vi "MBUS_U8toU16.vi"(11 "inputData":u8[](array[numeric])) -> (2 "ModbusExceptionCode":u8, 3 "outputData":u16[](array[numeric]))   [LabVIEW 2012, in "MBUS_Modbus.lvlib"]
uses:
  MBUS_Modbus.lvlib
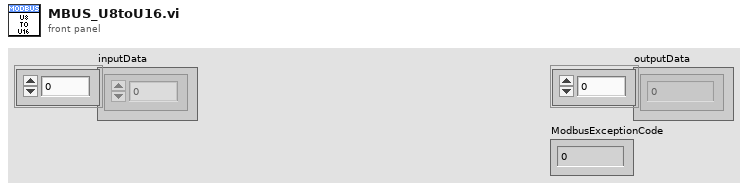
[diagram p1: front panel]
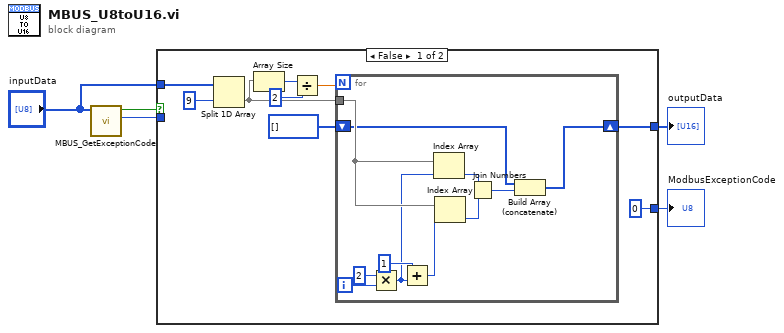
[diagram p0: block diagram]
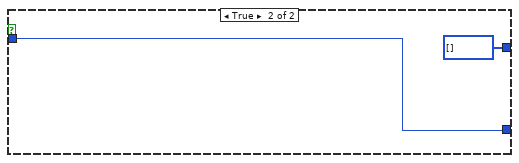
[diagram p2: hidden frame]
diagram:
  n1 = call "MBUS_GetExceptionCode.vi"("inputData"="inputData") -> ("ModbusExceptionCode"=w4:u8, "ModbusException"=w5:bool)  [unwired: 9 in]
  n2 = case shown="False" w5 {
    tunnel: w4 -> [_ w26]
    tunnel: "inputData" -> [w14 _]
    tunnel: [w11 u16[] []] -> w2
    tunnel: [u8 0 ("ModbusExceptionCode") w26] -> w1
    frame False {
      n3 = Split 1D Array(array=w14, index=9) -> (second subarray=w9:u8[])  [unwired: 1 out]
      n4 = Array Size(array=w9) -> (size(s)=w8:i32)
      n5 = Divide(x=w8, y=2) -> (x/y=w6:dbl)
      n6 = for {
        N: w6 -> [_]
        tunnel: w9 -> [w25]
        shift-right: [w21] -> w11
        shift-left: u16[] [] -> [w20]
        i -> [w19]
        n7 = Multiply(x=2, y=w19) -> (x*y=w16:i32)
        n8 = Add(x=1, y=w16) -> (x+y=w15:i32)
        n9 = Index Array(array=w25, index=w16) -> (element=w24:u8)
        n10 = Index Array(array=w25, index=w15) -> (element=w23:u8)
        n11 = Join Numbers(hi=w24, lo=w23) -> ((hi.lo)=w22:u16)
        n12 = Build Array (concatenate)(w20, w22) -> (w21:u16[])
      }
    }
    frame True {
    }
  }
  "outputData" <- w2
  "ModbusExceptionCode" <- w1
